vi "PH_ImageStatistician.export Data.vi"(0 "i ref in":refnum<vi>, 5 "error in (no error)":errorcluster) -> (14 "i ref out":refnum<vi>, 19 "error out":errorcluster)   [LabVIEW 2014, in "PH_ImageStatistician.lvlib"]
doc: "This VI exports data to a file"
uses:
  PH_ImageStatistician.lvlib
  PH_Common/PH_Common.lvlib
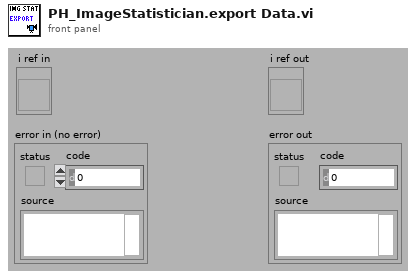
[diagram p1: front panel]
types:
  T1 = typedef "PH_ImageStatistician.lvlib/PH_ImageStatistician.i attribute.ctl" = cluster{"GUI Refs ":cluster{"Status":refnum<vi>, "Result Graph":refnum<vi>, "Mean Data 1":refnum<vi>, "Std Dev Data 1":refnum<vi>, "Mean Data 2":refnum<vi>, "Std Dev Data 2":refnum<vi>, "Mean Data 3":refnum<vi>, "Std Dev Data 3":refnum<vi>, "Dummy Mean":refnum<vi>, "Dummy Std Dev":refnum<vi>, "Export Data":refnum<vi>, "Data 1":refnum<vi>, "Data 2":refnum<vi>, "Data 3":refnum<vi>, "Stat or Trend":refnum<vi>, "Delete":refnum<vi>, "Operator":refnum<vi>, "Start":refnum<vi>}, "Operator":string, "Data":T2[], "Stat or Trend":bool, "Data 1":T3, "Data 2":T3, "Data 3":T3, "Start":bool, "Datasets strored":i32, "Dataarray Size":i32}
  T2 = typedef "PH_ImageStatistician.lvlib/PH_ImageStatistician.Statistician Data.ctl" = cluster{"Snapshot Time":dbl, "Maj FWHM":dbl, "Min FWHM":dbl, "Maj Fit Order":dbl, "Min Fit Order":dbl, "99% Diam Maj Trace":dbl, "99% Diam Min Trace":dbl, "Theta":dbl, "Delta":dbl, "Maj Diam":dbl, "Min Diam":dbl, "Azimuth Angle":dbl, "Azi Angle rel to major?":dbl, "Ellipticity":dbl, "CoG - X":dbl, "CoG - Y":dbl, "Energy":dbl, "Energy Cal - no mJ":dbl, "Lin Cal - no mm or mrad":dbl, "Lin Cal Factor":dbl}
  T3 = typedef "PH_ImageStatistician.lvlib/PH_ImageStatistician.select Data.ctl" = u16
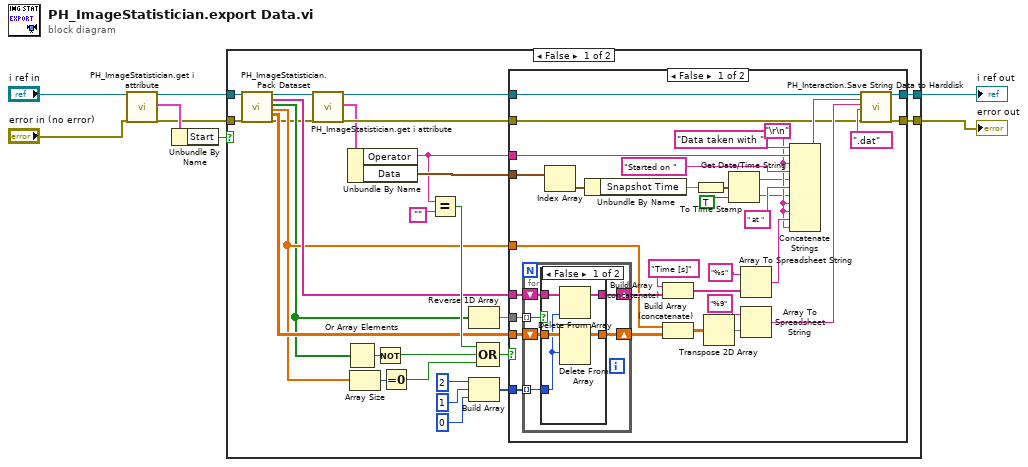
[diagram p0: block diagram]
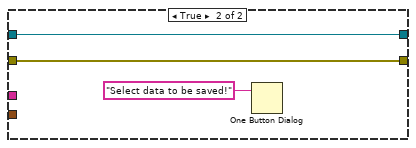
[diagram p3: hidden frame]
diagram:
  n1 = call "PH_ImageStatistician.get i attribute.vi"("i ref in"="i ref in", "error in (no error)"="error in (no error)") -> ("i ref out"=w2:refnum<vi>, "i attribute"=w6:T1, "error out"=w4:errorcluster)  [unwired: 15 in]
  n2 = Unbundle By Name(w6) -> ("Start"=w3:bool)
  n3 = case shown="False" w3 {
    tunnel: [w28 w86] -> w5
    tunnel: w4 -> [w17 w86]
    tunnel: w2 -> [w16 w85]
    tunnel: [w18 w85] -> w1
    frame False {
      n4 = call "PH_ImageStatistician.Pack Dataset.vi"("i ref in"=w16, "error in"=w17) -> ("i ref out"=w15:refnum<vi>, "Dataset Legend"=w27:string[], "Dataset chosen?"=w19:bool[], "Timebase"=w25:dbl[], "Dataset"=w26:dbl[][], "error out"=w13:errorcluster)  [unwired: 12 in]
      n5 = call "PH_ImageStatistician.get i attribute.vi"("i ref in"=w15, "error in (no error)"=w13) -> ("i ref out"=w14:refnum<vi>, "i attribute"=w11:T1, "error out"=w12:errorcluster)  [unwired: 15 in]
      n6 = Or Array Elements(Boolean array=w19) -> (logical OR=w34:bool)
      n7 = Unbundle By Name(w11) -> ("Operator"=w9:string, "Data"=w10:T2[])
      n8 = Array Size(array=w25) -> (size(s)=w30:i32)
      n9 = Not(x=w34) -> (.not. x?=w33:bool)
      n10 = Equal To 0?(x=w30) -> (x = 0?=w29:bool)
      n11 = Equal?(x=w9, y="") -> (x = y?=w32:bool)
      n12 = Reverse 1D Array(array=w19) -> (reversed array=w20:bool[])
      n13 = Build Array(2, 1, 0) -> (w21:i32[])
      n14 = Compound Arithmetic op=OR(w32, w33, w29) -> (w31:bool)
      n15 = case shown="False" w31 {
        tunnel: w9 -> [w64 _]
        tunnel: w27 -> [w60 _]
        tunnel: w26 -> [w58 _]
        tunnel: w20 -> [w59 _]
        tunnel: w12 -> [w46 w83]
        tunnel: [w45 w83] -> w28
        tunnel: w25 -> [w54 _]
        tunnel: w21 -> [w51 _]
        tunnel: w14 -> [w44 w82]
        tunnel: [w43 w82] -> w18
        tunnel: w10 -> [w36 _]
        frame False {
          w61 = "\r\n"
          n16 = for {
            tunnel: w59 -> [w70] mode=indexing
            shift-right: [w73] -> w56
            shift-left: w60 -> [w74]
            shift-right: [w71] -> w53
            shift-left: w58 -> [w72]
            tunnel: w51 -> [w69] mode=indexing
            n17 = case shown="False" w70 {
              tunnel: w74 -> [w79 w81]
              tunnel: [w78 w81] -> w73
              tunnel: w72 -> [w77 w80]
              tunnel: [w76 w80] -> w71
              tunnel: w69 -> [w75 _]
              frame False {
                n18 = Delete From Array(array=w79, index=w75) -> (array with subset deleted=w78:string[])  [unwired: 1 in, 1 out]
                n19 = Delete From Array(array=w77, index (row)=w75) -> (array with subset deleted=w76:dbl[][])  [unwired: 2 in, 1 out]
              }
              frame True {
              }
            }
          }
          n20 = Index Array(array=w36) -> (element=w37:T2)  [unwired: 1 in]
          n21 = Unbundle By Name(w37) -> ("Snapshot Time"=w38:dbl)
          n22 = Build Array (concatenate)("Time [s]" ("element"), w56) -> (w55:string[])
          n23 = Build Array (concatenate)(w54, w53) -> (w52:dbl[][])
          n24 = To Time Stamp(1:w38) -> (0:w39:timestamp)
          n25 = Transpose 2D Array(2D array=w52) -> (transposed array=w57:dbl[][])
          n26 = Get Date/Time String(seconds (now)=w39, want seconds? (F)=TRUE) -> (date string=w41:string, time string=w40:string)  [unwired: 1 in]
          n27 = Array To Spreadsheet String(array=w55, 3:"%s" ("format string")) -> (spreadsheet string=w62:string)  [unwired: 1 in]
          n28 = Array To Spreadsheet String(array=w57, 3:"%9" ("format string")) -> (spreadsheet string=w49:string)  [unwired: 1 in]
          n29 = Concatenate Strings("Data taken with " ("string"), w64, w61, "Started on ", w41, " at " ("string"), w40, w61, w61, w62, w61) -> (w47:string)
          n30 = call "PH_Interaction.Save String Data to Harddisk.vi"("i ref in"=w44, "Explanation (for Example: Column 1: xxx, ...)"=w47, "Data (for example: Columns)"=w49, "file name extension"=".dat" ("file name extinction"), "error in (no error)"=w46) -> ("i ref out"=w43:refnum<vi>, "error out"=w45:errorcluster)  [unwired: 12 in, 1 out]
        }
        frame True {
          n31 = One Button Dialog(message="Select data to be saved!") -> ()  [unwired: 1 in, 1 out]
        }
      }
    }
    frame True {
    }
  }
  "error out" <- w5
  "i ref out" <- w1
